vi "CB Local Sense Command and Read.vi"(7 "Board Selector":T1, 8 "error in (no error)":errorcluster, 9 "Message IN":string, 10 "Relay Control":bool[](array[boolean])) -> (0 "error out":errorcluster, 1 "Message OUT":string, 2 "Voltage Array":dbl[](array[numeric]), 3 "Control Board OUT":refnum<visa-resource-name>)   [LabVIEW 2022 SP3]
uses:
  Serial Board Com/Board Select.ctl
  Serial Board Com/ADCSelector BB.ctl
  Serial Board Com/ADCSelector GB.ctl
  <vilib>/DAQmx/write.llb/DAQmx Write (Digital 1D Bool NChan 1Samp 1Line).vi
  <vilib>/DAQmx/miscellaneous.llb/DAQmx Fill In Error Info.vi
panel:
  out "Vline_ca":dbl
  out "Vline_ab":dbl
  out "Vline_bc":dbl
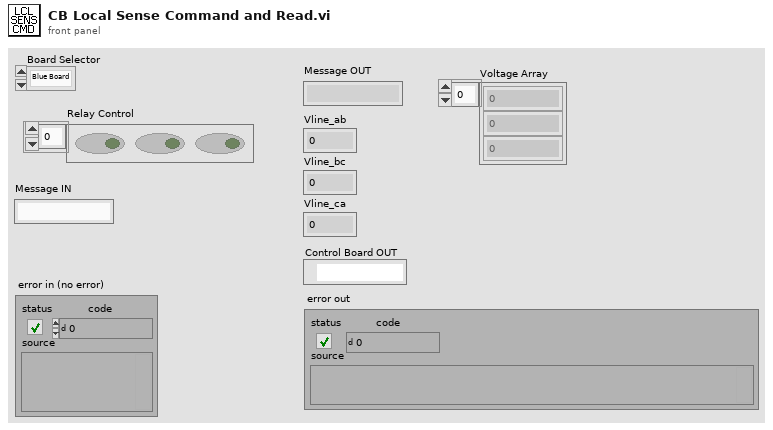
[diagram p1: front panel]
types:
  T1 = typedef "Board Select.ctl" = enum16{"Blue Board", "Green Board"}
  T2 = typedef "ADCSelector GB.ctl" = enum16{"INVA_ISENSE_U", "INVA_ISENSE_V", "INVA_ISENSE_W", "INVA_UDC", "INVA_TEMP", "HB_ISENSE", "AUX_ISENSE_U", "AUX_ISENSE_V", "AUX_ISENSE_W", "VLINE_AB", "VLINE_BC", "VLINE_CA", "REF_1P5V", "VSENSE_POS_24V", "VSENSE_POS_5V", "VSENSE_NEG_15V", "TEST_POINT", "INVB_ISENSE_U", "INVB_ISENSE_V", "INVB_ISENSE_W", "INVB_UDC", "INVB_TEMP", "HB_TEMP", "AUXA_TEMP", "AUXB_TEMP", "AUXC_TEMP", "VOUT_AB", "VOUT_BC", "VOUT_CA", "REF_2P5V", "VSENSE_POS_15V", "VSENSE_POS_3P3V", "NET_ANALYZER"}
  T3 = typedef "ADCSelector BB.ctl" = enum16{"INVA_ISENSE_U", "INVA_ISENSE_V", "INVA_ISENSE_W", "INVA_UDC", "INVA_TEMP", "HB_TEMP", "AUXB_TEMP", "VLINE_AB", "VLINE_BC", "VLINE_CA", "VSENSE_POS_24V", "VSENSE_POS_5V", "VSENSE_NEG_15V", "INVB_ISENSE_U", "INV_B_ISENSEV", "INVB_ISENSE_W", "INVB_UDC", "INVB_TEMP", "AUXA_TEMP", "AUXC_TEMP", "VOUT_AB", "VOUT_BC", "VOUT_CA", "VSENSE_POS_15V", "VSENSE_POS_3P3V", "TEST_POINT"}
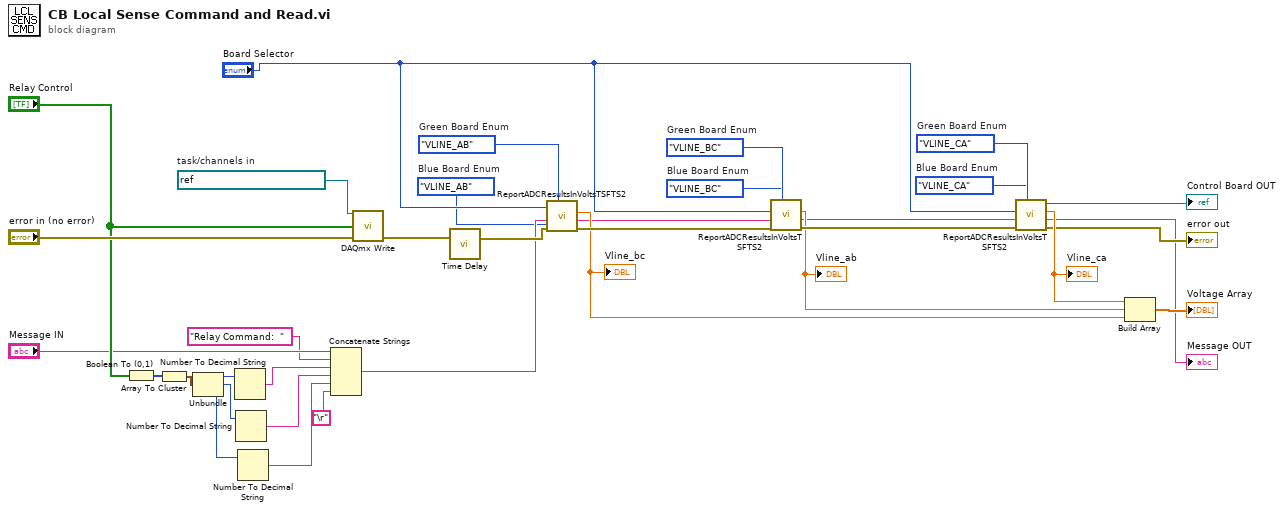
[diagram p0: block diagram]
diagram:
  w5 = ADCSelector_GB."VLINE_CA"  # Green Board Enum
  w6 = ADCSelector_GB."VLINE_BC"  # Green Board Enum
  w7 = ADCSelector_GB."VLINE_AB"  # Green Board Enum
  w32 = refnum<k21> "FTS2_LocalSenseRelays"  # task/channels in
  w1 = ADCSelector_BB."VLINE_CA"  # Blue Board Enum
  w2 = ADCSelector_BB."VLINE_BC"  # Blue Board Enum
  w3 = ADCSelector_BB."VLINE_AB"  # Blue Board Enum
  n1 = Boolean To (0,1)(Boolean="Relay Control") -> (0, 1=w22:i16[])
  n2 = Array To Cluster(array=w22) -> (cluster=w21:cluster{"[0]":i16, "[1]":i16, "[2]":i16})
  n3 = Unbundle(w21) -> ("[0]"=w20:i16, "[1]"=w19:i16, "[2]"=w18:i16)
  n4 = Number To Decimal String(number=w20) -> (decimal integer string=w15:string)  [unwired: 1 in]
  n5 = Number To Decimal String(number=w19) -> (decimal integer string=w16:string)  [unwired: 1 in]
  n6 = Number To Decimal String(number=w18) -> (decimal integer string=w17:string)  [unwired: 1 in]
  n7 = Concatenate Strings("Message IN", "Relay Command:  ", w15, w16, w17, "\r") -> (w14:string)
  n8 = call-poly <vilib>:"DAQmx Write.vi"("task/channels in"=w32, "data"="Relay Control", "error in"="error in (no error)") -> ("error out"=w33:errorcluster)  [unwired: 10 in, 2 out]
  n9 = call "Time Delay"("error in (no error)"=w33) -> ("error out"=w30:errorcluster)  [unwired: 10 in]
  n10 = call "ReportADCResultsInVoltsTSFTS2.vi"("Blue Board Enum"=w3, "Green Board Enum"=w7, "error in (no error)"=w30, "Message IN"=w14, "Board Selector"="Board Selector") -> ("error out"=w35:errorcluster, "Message OUT"=w13:string, "Result"=w27:dbl)  [unwired: 3 in, 1 out]
  "Vline_bc" <- w27
  n11 = call "ReportADCResultsInVoltsTSFTS2.vi"("Blue Board Enum"=w2, "Green Board Enum"=w6, "error in (no error)"=w35, "Message IN"=w13, "Board Selector"="Board Selector") -> ("error out"=w34:errorcluster, "Message OUT"=w12:string, "Result"=w29:dbl)  [unwired: 3 in, 1 out]
  "Vline_ab" <- w29
  n12 = call "ReportADCResultsInVoltsTSFTS2.vi"("Blue Board Enum"=w1, "Green Board Enum"=w5, "error in (no error)"=w34, "Message IN"=w12, "Board Selector"="Board Selector") -> ("error out"=→"error out":errorcluster, "Message OUT"=→"Message OUT":string, "Result"=w28:dbl, "VISA Refnum out"=→"Control Board OUT":refnum<visa-resource-name>)  [unwired: 3 in]
  "Vline_ca" <- w28
  n13 = Build Array(w28, w29, w27) -> (→"Voltage Array":dbl[])
